vi "Check Status.vi"(8 "error in":errorcluster, 11 "module handle":u32) -> (0 "error out":errorcluster, 2 "status values":dbl[](array[numeric]), 3 "module handle out":u32)   [LabVIEW 2020, in "AIM MIL-STD-1553 Hardware API.lvlib"]
uses:
  AIM MIL-STD-1553 Hardware API.lvlib
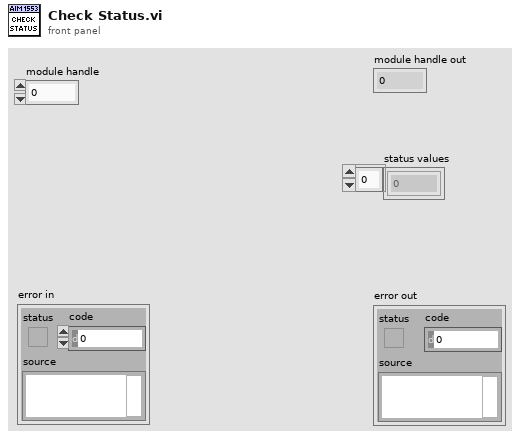
[diagram p1: front panel]
types:
  T1 = cluster{"Status Trigger Pattern":u8, "Global Message Count":u32, "Global Error Count":u32}
  T2 = cluster{"Global Word Count":u32, "Global Message Count":u32, "Global Error Count":u32, "Current Bus Load %":dbl, "Average Bus Load %":dbl}
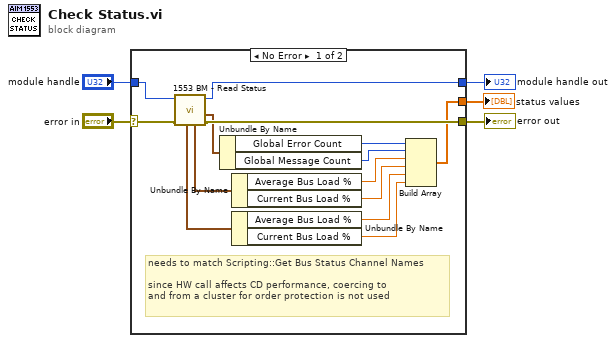
[diagram p0: block diagram]
diagram:
  n1 = case shown="No Error" "error in" {
    selector: "error in" -> [w19 w22]
    tunnel: [w18 w22] -> w5
    tunnel: "module handle" -> [w14 w21]
    tunnel: [w13 w21] -> w2
    tunnel: [w6 dbl[] []] -> w1
    frame No Error {
      # "needs to match Scripting::Get Bus Status Channel Names\n\nsince HW call affects CD performance, coercing to \nand from a cluster for order protection is not used"
      n2 = call <instrlib>:"1553 BM - Read Status.vi"("Error In (none)"=w19, "Module Handle"=w14) -> ("Error Out"=w18:errorcluster, "Global Counts"=w15:T1, "Module Handle Out"=w13:u32, "Primary Bus"=w17:T2, "Secondary Bus"=w16:T2)  [unwired: 4 in, 1 out]
      n3 = Unbundle By Name(w15) -> ("Global Error Count"=w7:u32, "Global Message Count"=w8:u32)
      n4 = Unbundle By Name(w17) -> ("Average Bus Load %"=w9:dbl, "Current Bus Load %"=w10:dbl)
      n5 = Unbundle By Name(w16) -> ("Average Bus Load %"=w11:dbl, "Current Bus Load %"=w12:dbl)
      n6 = Build Array(w7, w8, w9, w10, w11, w12) -> (w6:dbl[])
    }
    frame Error {
    }
  }
  "error out" <- w5
  "module handle out" <- w2
  "status values" <- w1
